vi "Read reference.vi"(8 "error in (no error)":errorcluster, 11 "MelsecMcNet in":refnum<class "MelsecMcNet.lvclass">) -> (0 "error out":errorcluster, 2 "reference":refnum<k24>, 3 "MelsecMcNet out":refnum<class "MelsecMcNet.lvclass">)   [LabVIEW 2020, in "HslCommunication.lvlib" / "MelsecMcNet.lvclass"]
uses:
  MelsecMcNet.lvclass
  E:/Git/Libraries/develop/PLCMonitor/HslCommunication/_Dependenciecs/HslCommunication.dll
  _Dependenciecs/HslCommunication.dll
  MelsecMcNet.lvclass/MelsecMcNet.ctl
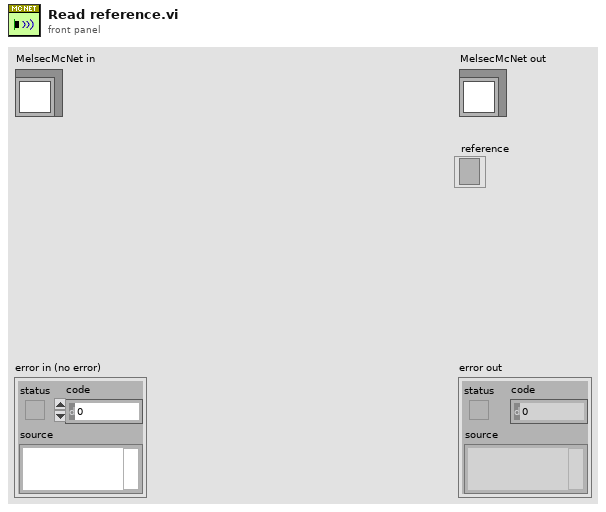
[diagram p1: front panel]
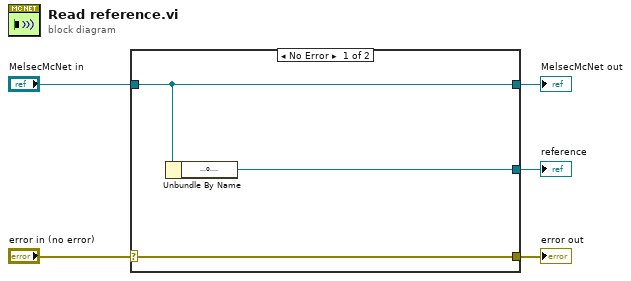
[diagram p0: block diagram]
diagram:
  n1 = case shown="No Error" "error in (no error)" {
    selector: "error in (no error)" -> [w8 w9]
    tunnel: [w8 w9] -> w4
    tunnel: [w7 w10] -> w2
    tunnel: "MelsecMcNet in" -> [w7 w10]
    tunnel: [w6 _] -> w1
    frame No Error {
      n2 = Unbundle By Name(w7) -> ("reference"=w6:refnum<k24>)
    }
    frame Error {
    }
  }
  "error out" <- w4
  "MelsecMcNet out" <- w2
  "reference" <- w1
